vi "SubVINode.vi"(1 "Path":path, 2 "Owner":refnum<vi>) -> (0 "Node":refnum<vi>)   [LabVIEW 2014]
uses:
  <vilib>/Utility/miscctls.llb/LVPointTypeDef.ctl
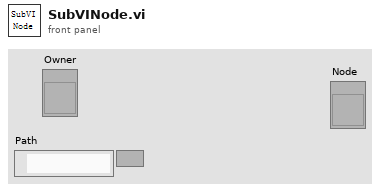
[diagram p1: front panel]
types:
  T1 = typedef "LVPointTypeDef.ctl" = cluster{"Horizontal":i16, "Vertical":i16}
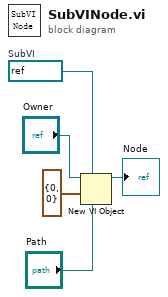
[diagram p0: block diagram]
diagram:
  w5 = refnum<vi> refnum  # SubVI
  n1 = New VI Object(vi object class=w5, owner refnum="Owner", position/next to=T1 {"Horizontal"=0, "Vertical"=0} ("location"), 6:"Path") -> (object refnum=→"Node":refnum<vi>)  [unwired: 4 in, 1 out]
